vi "Read RD Error.vi"(4 "error in (no error)":errorcluster, 6 "Container State":T2, 7 "Display State In":T1) -> (0 "error out":errorcluster, 2 "Value":bool, 3 "Display State Out":T1)   [LabVIEW 2015, in "Ringdown.xctl"]
uses:
  Ringdown.xctl
  <vilib>/_xctls/Container State.ctl
  Ringdown State.ctl
  <vilib>/_xctls/XControlSupport.lvlib
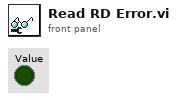
[diagram p1: front panel]
types:
  T1 = typedef "Ringdown.xctl/Ringdown State.ctl" = cluster{"Dispaly Data":bool, "Display Fit":bool, "Trace":bool[], "RD Error ":bool, "Display Random":bool}
  T2 = typedef "XControlSupport.lvlib/Container State.ctl" = cluster{"Indicator?":bool, "Run Mode?":bool, " Refnum":refnum<vi>}
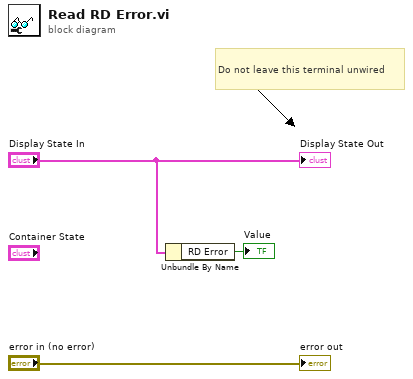
[diagram p0: block diagram]
diagram:
  # "Do not leave this terminal unwired"
  n1 = Unbundle By Name("Display State In") -> ("RD Error"=→"Value":bool)
  "error out" <- "error in (no error)"
  "Display State Out" <- "Display State In"
